vi "Format Queue Service Properties.vi"(11 "Queue service properties":T1) -> (3 "Queue service string":string)   [LabVIEW 2015, in "NI_Azure_Queue.lvlib"]
uses:
  NI_Azure_Queue.lvlib
  Queue Service Properties.ctl
  Logging.ctl
  Retention Policy.ctl
  Metrics.ctl
  Cors Rule.ctl
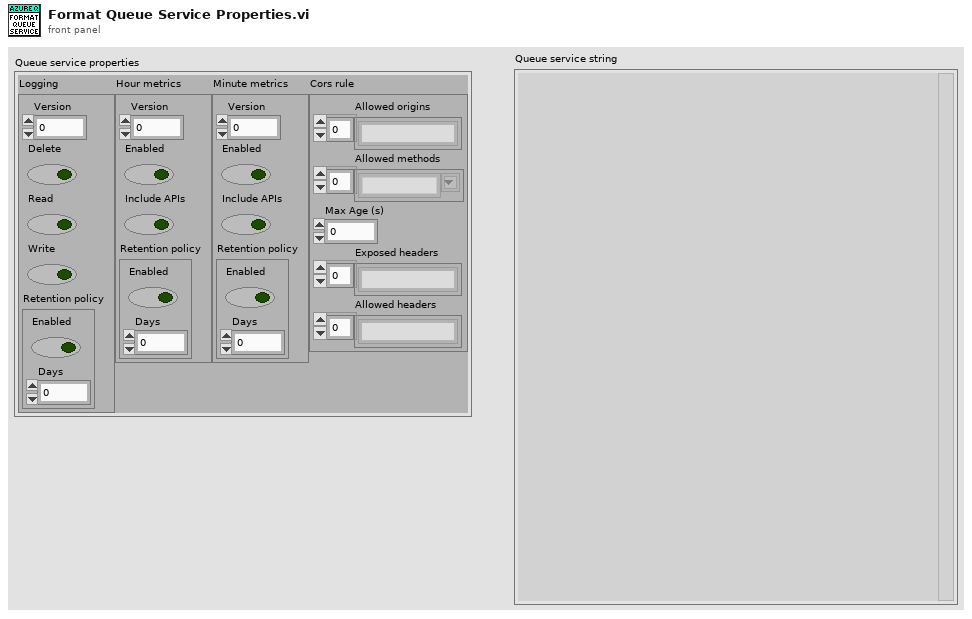
[diagram p1: front panel]
types:
  T1 = typedef "NI_Azure_Queue.lvlib/Queue Service Properties.ctl" = cluster{"Logging":T2, "Hour metrics":T4, "Minute metrics":T4, "Cors rule":T5}
  T2 = typedef "NI_Azure_Queue.lvlib/Logging.ctl" = cluster{"Version":dbl, "Delete":bool, "Read":bool, "Write":bool, "Retention policy":T3}
  T3 = typedef "NI_Azure_Queue.lvlib/Retention Policy.ctl" = cluster{"Enabled":bool, "Days":u32}
  T4 = typedef "NI_Azure_Queue.lvlib/Metrics.ctl" = cluster{"Version":dbl, "Enabled":bool, "Include APIs":bool, "Retention policy":T3}
  T5 = typedef "NI_Azure_Queue.lvlib/Cors Rule.ctl" = cluster{"Allowed origins":string[], "Allowed methods":string[], "Max Age (s)":u32, "Exposed headers":string[], "Allowed headers":string[]}
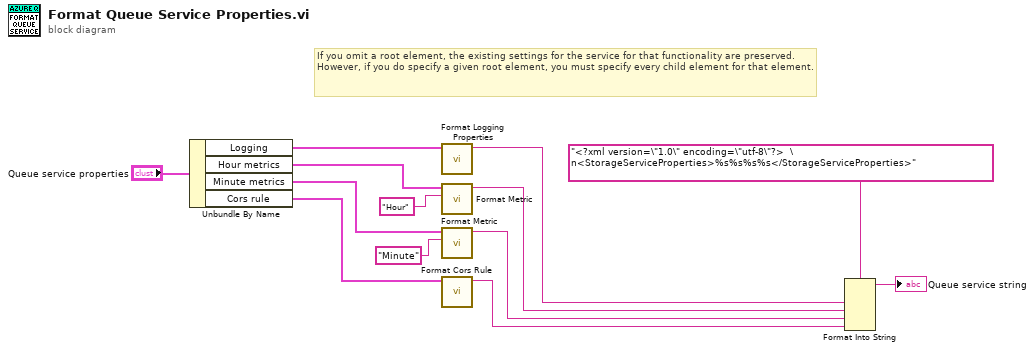
[diagram p0: block diagram]
diagram:
  # "If you omit a root element, the existing settings for the service for that functionality are preserved. However, if you do specify a given root element, you must specify every child element for that element."
  n1 = Unbundle By Name("Queue service properties") -> ("Logging"=w12:T2, "Hour metrics"=w9:T4, "Minute metrics"=w8:T4, "Cors rule"=w2:T5)
  n2 = call "Format Logging Properties.vi"("Logging properties"=w12) -> ("Logging string"=w6:string)  [unwired: 10 in]
  n3 = call "Format Metric.vi"("Metric name"="Hour", "Metric properties"=w9) -> ("Metrics string"=w5:string)  [unwired: 9 in]
  n4 = call "Format Metric.vi"("Metric name"="Minute", "Metric properties"=w8) -> ("Metrics string"=w4:string)  [unwired: 9 in]
  n5 = call "Format Cors Rule.vi"("Cors rule"=w2) -> ("Cors rule string"=w1:string)  [unwired: 10 in]
  n6 = Format Into String(format string="<?xml version=\"1.0\" encoding=\"utf-8\"?>  \n<StorageServiceProperties>%s%s%s%s</StorageServiceProperties>", w6, w5, w4, w1) -> (resulting string=→"Queue service string":string)  [unwired: 2 in, 1 out]
